vi "DAG size.vi"(9 "DAG in":refnum<class "DAG.lvclass">) -> (3 "DAG out":refnum<class "DAG.lvclass">, 4 "edges":i32, 5 "vertices":i32)   [LabVIEW 2014, in "Raspberry Pi Compatible Compiler for LabVIEW.lvlib" / "DAG.lvclass"]
uses:
  DAG.lvclass
  DAG.lvclass/DAG.ctl
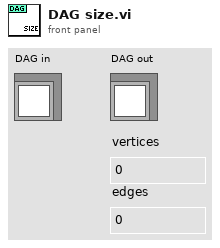
[diagram p1: front panel]
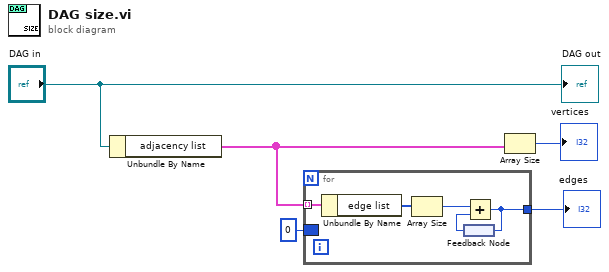
[diagram p0: block diagram]
diagram:
  n1 = Unbundle By Name("DAG in") -> ("adjacency list"=w4:cluster{"edge list":i32[]}[])
  n2 = for {
    tunnel: w4 -> [w10] mode=indexing
    tunnel: [w6] -> w2
    border: 0 -> [_]
    n3 = Unbundle By Name(w10) -> ("edge list"=w9:i32[])
    n4 = Array Size(array=w9) -> (size(s)=w8:i32)
    n5 = feedback #1() -> (w7:i32)
    n6 = Add(x=w8, y=w7) -> (x+y=w6:i32)
    n7 = feedback-in #1(w6) -> ()
  }
  "edges" <- w2
  n8 = Array Size(array=w4) -> (size(s)=→"vertices":i32)
  "DAG out" <- "DAG in"
